vi "Save Files for Previous Version.vi"(8 "error in (no error)":errorcluster, 10 "LabVIEW Files to Convert":path[](array[path]), 11 "Session in":refnum<class "Session.lvclass">) -> (0 "error out":errorcluster, 3 "Session out":refnum<class "Session.lvclass">)   [LabVIEW 2020, in "Save for Previous Version.lvlib" / "Session.lvclass"]
uses:
  Session.lvclass
  Session.lvclass/Session.ctl
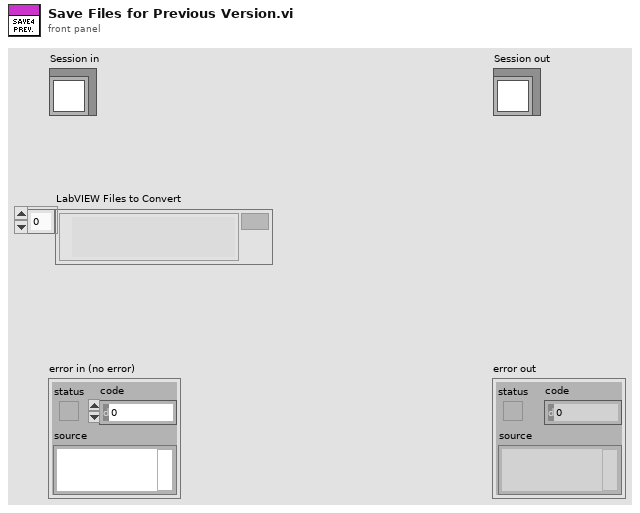
[diagram p1: front panel]
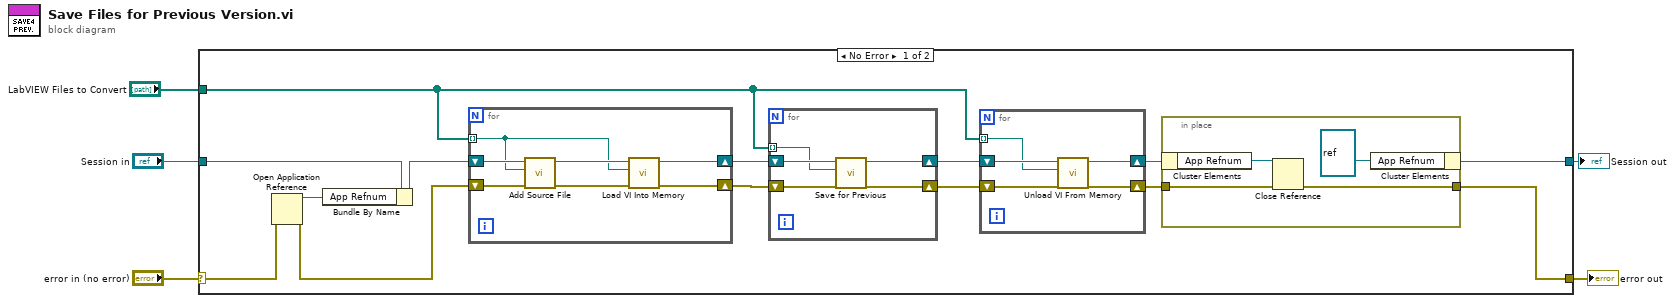
[diagram p0: block diagram]
diagram:
  n1 = case shown="No Error" "error in (no error)" {
    selector: "error in (no error)" -> [w11 w42]
    tunnel: [w6 w42] -> w4
    tunnel: [w8 w41] -> w2
    tunnel: "Session in" -> [w13 w41]
    tunnel: "LabVIEW Files to Convert" -> [w15 _]
    frame No Error {
      n2 = Open Application Reference(8:w11) -> (0:w10:errorcluster, 3:w12:refnum<vi>)  [unwired: 3 in]
      n3 = Bundle By Name(cluster=w13, "App Refnum"=w12) -> (w14:refnum<class "Session.lvclass">)
      n4 = for {
        tunnel: w15 -> [w34] mode=indexing
        shift-right: [w35] -> w17
        shift-left: w14 -> [w40]
        shift-right: [w37] -> w19
        shift-left: w10 -> [w39]
        n5 = call "Add Source File.vi"("error in (no error)"=w39, "Source File"=w34, "Session in"=w40) -> ("error out"=w38:errorcluster, "Session out"=w36:refnum<class "Session.lvclass">)  [unwired: 7 in]
        n6 = call "Load VI Into Memory.vi"("error in (no error)"=w38, "VI Path"=w34, "Session in"=w36) -> ("error out"=w37:errorcluster, "Session out"=w35:refnum<class "Session.lvclass">)  [unwired: 7 in]
      }
      n7 = for {
        shift-right: [w24] -> w18
        shift-left: w19 -> [w28]
        shift-right: [w26] -> w16
        shift-left: w17 -> [w27]
        tunnel: w15 -> [w25] mode=indexing
        n8 = call "Save for Previous.vi"("error in (no error)"=w28, "File Path"=w25, "Session in"=w27) -> ("error out"=w24:errorcluster, "Session out"=w26:refnum<class "Session.lvclass">)  [unwired: 7 in]
      }
      n9 = for {
        shift-right: [w31] -> w7
        shift-left: w18 -> [w32]
        tunnel: w15 -> [w30] mode=indexing
        shift-right: [w29] -> w9
        shift-left: w16 -> [w33]
        n10 = call "Unload VI From Memory.vi"("error in (no error)"=w32, "VI Path"=w30, "Session in"=w33) -> ("error out"=w31:errorcluster, "Session out"=w29:refnum<class "Session.lvclass">)  [unwired: 7 in]
      }
      n11 = in-place {
        in-place-border: w7 -> [w21]
        in-place-border: [w20] -> w6
        n12 = in-place-cluster #1(w9) -> ("App Refnum"=w23:refnum<vi>)
        n13 = Close Reference(reference=w23, error in (no error)=w21) -> (error out=w20:errorcluster)
        n14 = in-place-cluster #1("App Refnum"=refnum<vi> refnum) -> (w8:refnum<class "Session.lvclass">)
      }
    }
    frame Error {
    }
  }
  "error out" <- w4
  "Session out" <- w2
